vi "Speed Convertor.vi"() -> ()   [LabVIEW 2023]
panel:
  out "Speed (km)":dbl
  out "Output String Indicator":string
  in  "Speed (miles)":sgl format="%#_6f"
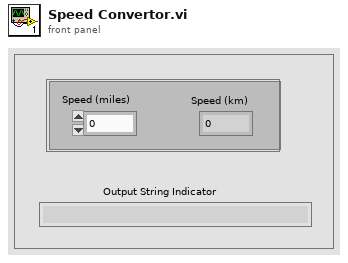
[diagram p1: front panel]
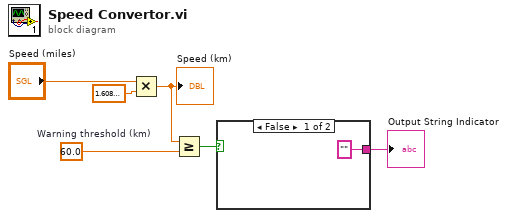
[diagram p0: block diagram]
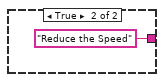
[diagram p2: hidden frame]
diagram:
  w3 = sgl 60.0  # Warning threshold (km)
  n1 = Multiply(x="Speed (miles)", y=sgl 1.609) -> (x*y=w4:sgl)
  "Speed (km)" <- w4
  n2 = Greater Or Equal?(x=w4, y=w3) -> (x >= y?=w1:bool)
  n3 = case shown="False" w1 {
    tunnel: ["" "Reduce the Speed"] -> w2
    frame False {
    }
    frame True {
    }
  }
  "Output String Indicator" <- w2
